vi "Tell.vi"(10 "Msg":refnum<class "Msg.lvclass">, 11 "Queue Transport in":refnum<class "Queue Transport.lvclass">) -> (0 "Error out":errorcluster)   [LabVIEW 2025, in "jettl.lvlib" / "Queue Transport.lvlib" / "Queue Transport.lvclass"]
uses:
  Queue Transport.lvclass
  Msg/Msg.lvclass
  Queue Transport.lvclass/Queue Transport.ctl
  Msg Input/Msg Input.lvclass
  Teller/Teller.lvclass
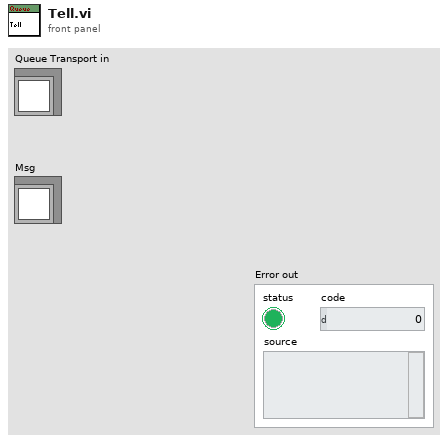
[diagram p1: front panel]
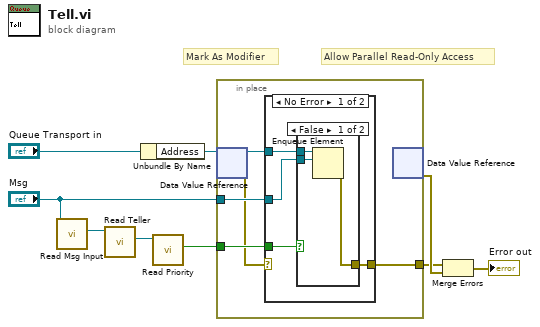
[diagram p0: block diagram]
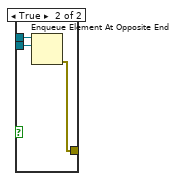
[diagram p2: hidden frame]
diagram:
  # "Allow Parallel Read-Only Access"
  # "Mark As Modifier"
  n1 = call-dynamic "Read Msg Input.vi"("Msg in"="Msg") -> ("Msg Input"=w2:refnum<class "Msg Input.lvclass">)  [unwired: 10 in]
  n2 = call-dynamic "Read Teller.vi"("Msg Input in"=w2) -> ("Teller"=w1:refnum<class "Teller.lvclass">)  [unwired: 10 in]
  n3 = Unbundle By Name("Queue Transport in") -> ("Address"=w8:refnum<data-value>)
  n4 = call-dynamic "Read Priority.vi"("Teller in"=w1) -> ("Priority"=w4:bool)  [unwired: 10 in]
  n5 = in-place {
    in-place-border: [w14] -> w5
    in-place-border: "Msg" -> [w13]
    in-place-border: w4 -> [w12]
    n6 = in-place-dvr #1(w8) -> (w11:refnum<queue>, w10:errorcluster)
    n7 = case shown="No Error" w10 {
      selector: w10 -> [_ w25]
      tunnel: [w18 w25] -> w14
      tunnel: w13 -> [w17 _]
      tunnel: w12 -> [w16 _]
      tunnel: w11 -> [w15 _]
      frame No Error {
        n8 = case shown="False" w16 {
          tunnel: w15 -> [w21 w24]
          tunnel: [w20 w22] -> w18
          tunnel: w17 -> [w19 w23]
          frame False {
            n9 = Enqueue Element(queue=w21, element=w19) -> (error out=w20:errorcluster)  [unwired: 2 in, 2 out]
          }
          frame True {
            n10 = Enqueue Element At Opposite End(queue=w24, element=w23) -> (error out=w22:errorcluster)  [unwired: 2 in, 2 out]
          }
        }
      }
      frame Error {
      }
    }
    n11 = in-place-dvr #1() -> (w6:errorcluster)  [unwired: 1 in, 1 out]
  }
  n12 = Merge Errors(w5, w6) -> (→"Error out":errorcluster)
